vi "ErrorDaemon.set.vi"(10 "ErrorHandler":refnum<class "ErrorHandler.lvclass">, 11 "TemplateDaemon in":refnum<class "MemoryManager.lvclass">) -> (3 "TemplateDaemon out":refnum<class "MemoryManager.lvclass">)   [LabVIEW 2024, in "MemoryManager.lvclass"]
uses:
  MemoryManager.lvclass
  MemoryManager.lvclass/MemoryManager.ctl
  ErrorHandler/ErrorHandler.lvclass
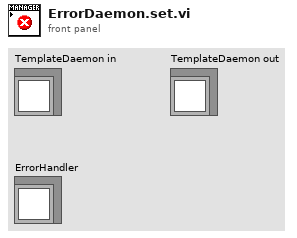
[diagram p1: front panel]
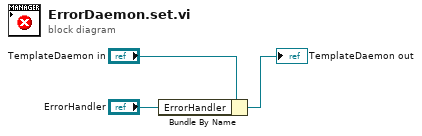
[diagram p0: block diagram]
diagram:
  n1 = Bundle By Name(cluster="TemplateDaemon in", "ErrorHandler"="ErrorHandler") -> (→"TemplateDaemon out":refnum<class "MemoryManager.lvclass">)
